vi "_Remote Single Update.vi"(4 "error in":errorcluster, 5 "DACValue":i32, 6 "ParamName":string, 7 "Running":bool) -> (0 "error out":errorcluster)   [LabVIEW 2012]
uses:
  Type/_RT Active Ch.ctl
  Type/_RT Command.ctl
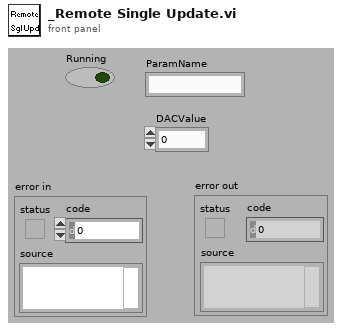
[diagram p1: front panel]
types:
  T1 = typedef "_RT Configuration 2.ctl" = cluster{"Name":string, "Ch#":u8, "Min":dbl, "Max":dbl, "Def+":dbl, "Def-":dbl, "Offset":dbl, "Slope":dbl, "Type":u8, "Description":string, "SettleT":dbl}
  T2 = typedef "_RT Active Ch.ctl" = cluster{"Start":i32, "Step":i32, "ChID":i32}
  T3 = typedef "_RT Command.ctl" = enum16{"Start", "Stop", "Runtime Update", "Get Data", "Get Info", "Get Status", "Get Param", "Get Config", "Get Table", "Read ADC", "Set Oscillator", "Update Config", "Update Table", "Set All Pol", "Set Pol and DC", "Set Max Mass", "Toggle RP", "Toggle EL", "Set PIC", "Initialize Turbo", "Send Turbo Comm", "Close Turbo", "P1", "P2", "P3", "Send Serial", "Set LC Out", "Get LC In", "Read VAC", "Test Table", "Toggle Power", "Get Startup", "Set Startup", "Get ADC Table", "Set ADC Table", "Get Brief Status", "Get Detail Status", "Auxiliary Update", "Set CC Logics", "Set CC Input Logics", "Ignore Error"}
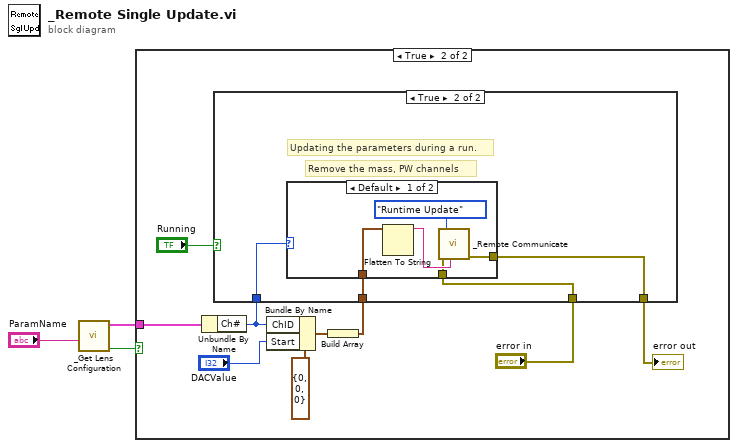
[diagram p0: block diagram]
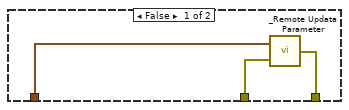
[diagram p3: hidden frame]
diagram:
  n1 = call "_Get Lens Configuration.vi"("Name"="ParamName") -> ("Found"=w1:bool, "Lens Configuration"=w2:T1)  [unwired: 1 in, 4 out]
  n2 = case shown="True" w1 {
    tunnel: w2 -> [_ w9]
    frame False {
    }
    frame True {
      n3 = Unbundle By Name(w9) -> ("Ch#"=w4:u8)
      n4 = Bundle By Name(cluster=T2 {"Start"=0, "Step"=0, "ChID"=0} ("Active Channel"), "ChID"=w4, "Start"="DACValue") -> (w5:T2)
      n5 = Build Array(w5) -> (w6:T2[])
      n6 = case shown="True" "Running" {
        tunnel: "error in" -> [w15 w16]
        tunnel: [w14 w17] -> w11
        tunnel: w6 -> [w13 w18]
        tunnel: w4 -> [_ w19]
        frame False {
          n7 = call "_Remote Updata Parameter.vi"("error in"=w15, "Parameters"=w13) -> ("error out"=w14:errorcluster)
        }
        frame True {
          # "Remove the mass, PW channels"
          # "Updating the parameters during a run."
          n8 = case shown="Default" w19 {
            tunnel: w18 -> [w24 _]
            tunnel: [w20 w25] -> w17
            tunnel: w16 -> [w21 w25]
            frame Default {
              n9 = Flatten To String(anything=w24) -> (data string=w22:string)  [unwired: 1 in, 4 out]
              n10 = call "_Remote Communicate.vi"("String"=w22, "error in (no error)"=w21, "Command"=_RT_Command."Runtime Update") -> ("error out"=w20:errorcluster)  [unwired: 3 in, 3 out]
            }
            frame 0..2, 4, 5, 7, 9 {
            }
          }
        }
      }
      "error out" <- w11
    }
  }
